vi "Sub_Preprocessing_FEA_Element_Matrix.vi"(1 "Length of Beam":dbl, 3 "Young's Modulus":dbl, 4 "No. of Nodes":i32, 5 "Height":dbl, 7 "Width":dbl, 10 "Density":dbl) -> (17 "Element Length":dbl, 18 "M Element Matrix":dbl[][](array[numeric]), 19 "K Element Matrix":dbl[][](array[numeric]))   [LabVIEW 2021]
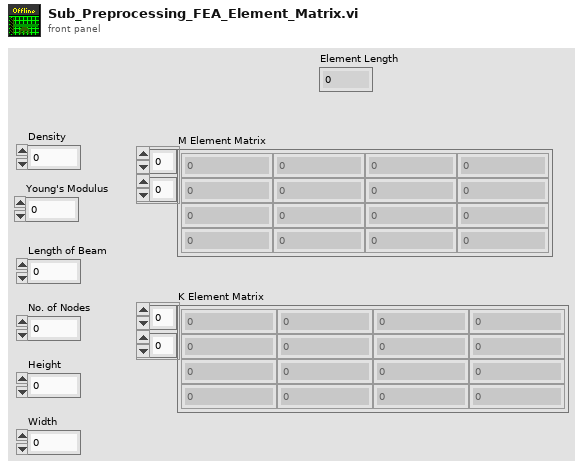
[diagram p1: front panel]
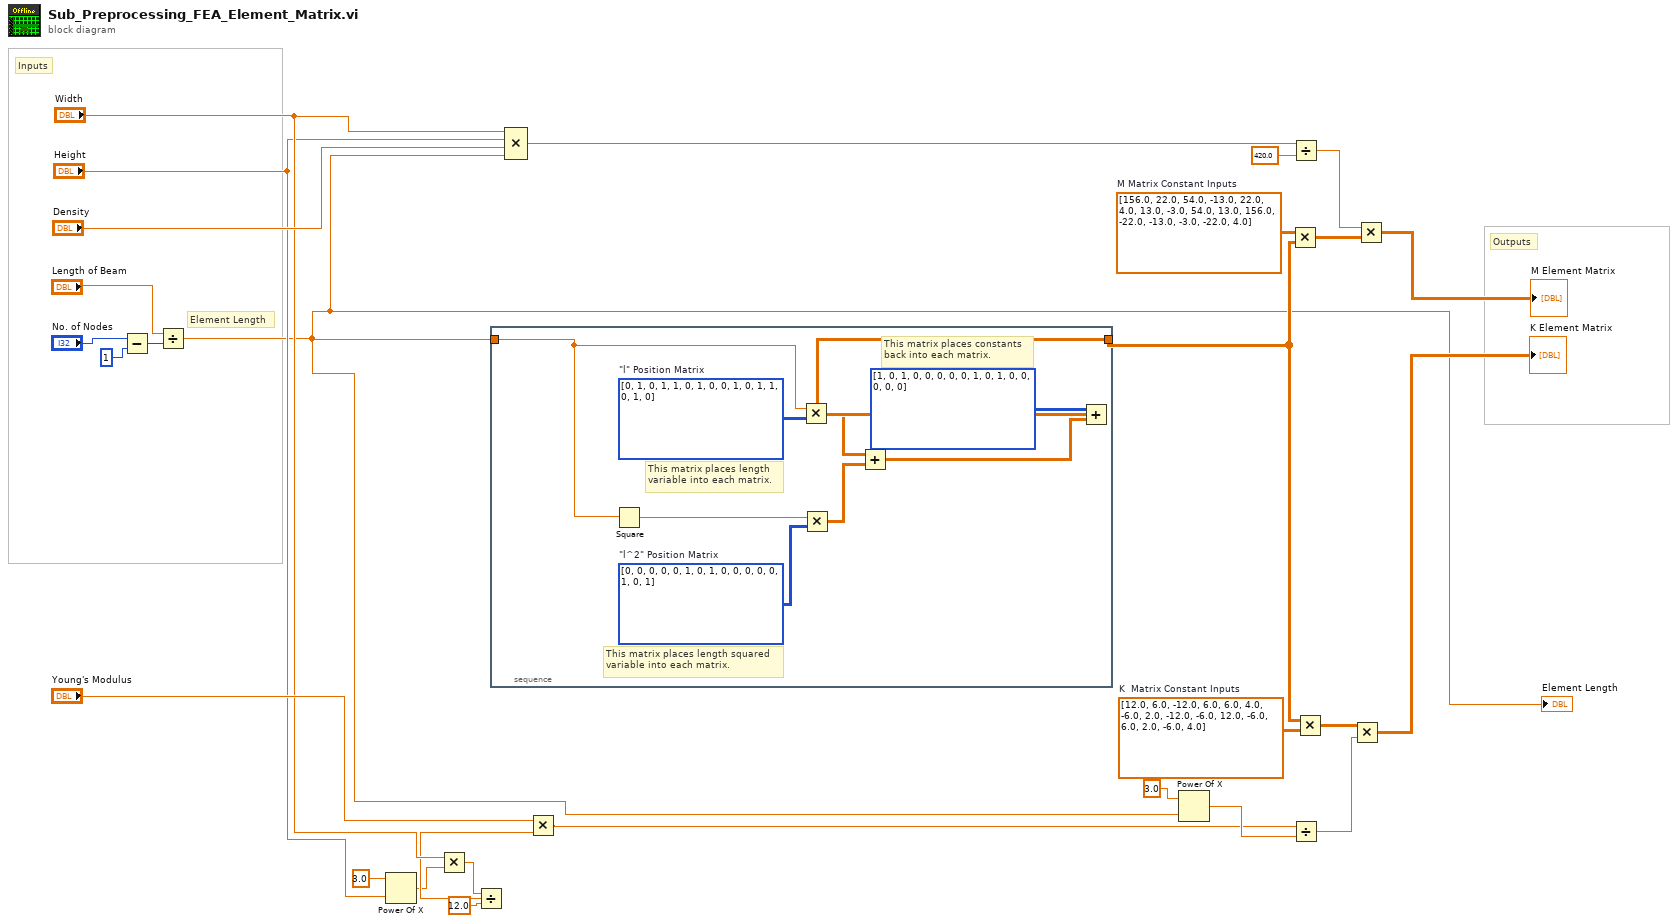
[diagram p0: block diagram]
diagram:
  w17 = dbl[][] [[12.0, 6.0, -12.0, 6.0], [6.0, 4.0, -6.0, 2.0], [-12.0, -6.0, 12.0, -6.0], [6.0, 2.0, -6.0, 4.0]]  # K  Matrix Constant Inputs
  w24 = dbl[][] [[156.0, 22.0, 54.0, -13.0], [22.0, 4.0, 13.0, -3.0], [54.0, 13.0, 156.0, -22.0], [-13.0, -3.0, -22.0, 4.0]]  # M Matrix Constant Inputs
  # "Outputs"
  # "Element Length"
  # "Inputs"
  n1 = Subtract(x="No. of Nodes", y=1) -> (x-y=w23:i32)
  n2 = Divide(x="Length of Beam", y=w23) -> (x/y=w6:dbl)
  "Element Length" <- w6
  n3 = Power Of X(1:"Height", 2:3.0 ("x")) -> (0:w3:dbl)
  n4 = Multiply(x="Width", y=w3) -> (x*y=w2:dbl)
  n5 = Divide(x=w2, y=12.0) -> (x/y=w8:dbl)
  n6 = stacked-sequence {
    tunnel: [w35] -> w18
    tunnel: w6 -> [w37]
    frame #0 {
      w30 = i32[][] [[0, 0, 0, 0], [0, 1, 0, 1], [0, 0, 0, 0], [0, 1, 0, 1]]  # "l^2" Position Matrix
      w29 = i32[][] [[0, 1, 0, 1], [1, 0, 1, 0], [0, 1, 0, 1], [1, 0, 1, 0]]  # "l" Position Matrix
      # "This matrix places length squared\nvariable into each matrix."
      # "This matrix places length \nvariable into each matrix."
      # "This matrix places constants\nback into each matrix."
      n7 = Square(x=w37) -> (x^2=w32:dbl)
      n8 = Multiply(x=w37, y=w29) -> (x*y=w31:dbl[][])
      n9 = Multiply(x=w32, y=w30) -> (x*y=w33:dbl[][])
      n10 = Add(x=w31, y=w33) -> (x+y=w36:dbl[][])
      n11 = Add(x=i32[][] [[1, 0, 1, 0], [0, 0, 0, 0], [1, 0, 1, 0], [0, 0, 0, 0]], y=w36) -> (x+y=w35:dbl[][])
    }
  }
  n12 = Compound Arithmetic op=MULTIPLY("Width", "Height", "Density", w6) -> (w26:dbl)
  n13 = Multiply(x="Young's Modulus", y=w8) -> (x*y=w11:dbl)
  n14 = Power Of X(1:w6, 2:3.0 ("x")) -> (0:w16:dbl)
  n15 = Multiply(x=w24, y=w18) -> (x*y=w27:dbl[][])
  n16 = Divide(x=w26, y=420.0) -> (x/y=w28:dbl)
  n17 = Divide(x=w11, y=w16) -> (x/y=w15:dbl)
  n18 = Multiply(x=w18, y=w17) -> (x*y=w14:dbl[][])
  n19 = Multiply(x=w14, y=w15) -> (x*y=→"K Element Matrix":dbl[][])
  n20 = Multiply(x=w28, y=w27) -> (x*y=→"M Element Matrix":dbl[][])
